vi "Teste Call.vi"(10 "FPS":dbl) -> ()   [LabVIEW 2022 SP3, in "Phoenix.lvclass"]
uses:
  Phoenix.lvclass
panel:
  out "current time":timestamp
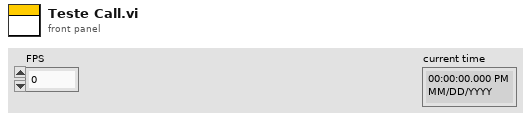
[diagram p1: front panel]
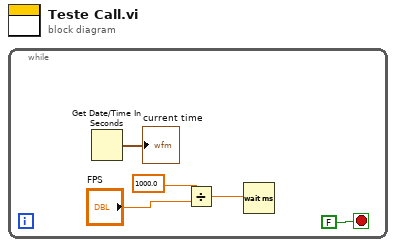
[diagram p0: block diagram]
diagram:
  n1 = while {
    stop <- FALSE stop-if-true
    n2 = Get Date/Time In Seconds() -> (seconds since 1Jan1904=→"current time":timestamp)
    n3 = Divide(x=1000.0, y="FPS") -> (x/y=w2:dbl)
    n4 = Wait (ms)(milliseconds to wait=w2) -> ()  [unwired: 1 out]
  }
